vi "sub_IR_data_buffer.vi"(7 "cmd":enum16{"write", "read"}(ring), 11 "IR data":i16[][](array[numeric])) -> (3 "IR data out":i16[][](array[numeric]))   [LabVIEW 2016]
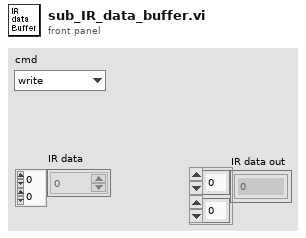
[diagram p1: front panel]
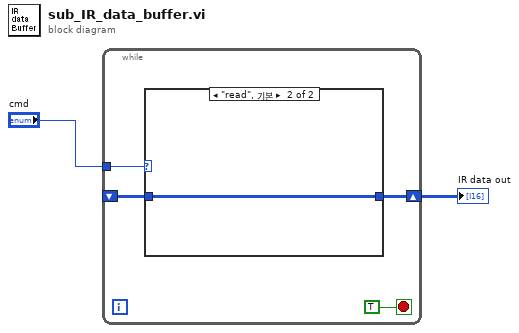
[diagram p0: block diagram]
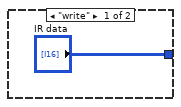
[diagram p2: hidden frame]
diagram:
  n1 = while {
    tunnel: "cmd" -> [w5]
    shift-right: [w4] -> w1
    shift-left: _ -> [w3]
    stop <- TRUE stop-if-true
    n2 = case shown="\"read\", 기본" w5 {
      tunnel: ["IR data" w8] -> w4
      tunnel: w3 -> [_ w8]
      frame "write" {
      }
      frame "read", Default {
      }
    }
  }
  "IR data out" <- w1
